vi "Generate Error.vi"(8 "Error In":errorcluster, 9 "Args":string[](array[string]), 10 "Nest Error":T1) -> (0 "Error Out":errorcluster)   [LabVIEW 2013, in "LVH-Nest.lvlib"]
uses:
  LVH-Nest.lvlib
  Type Defs/Nest Error.ctl
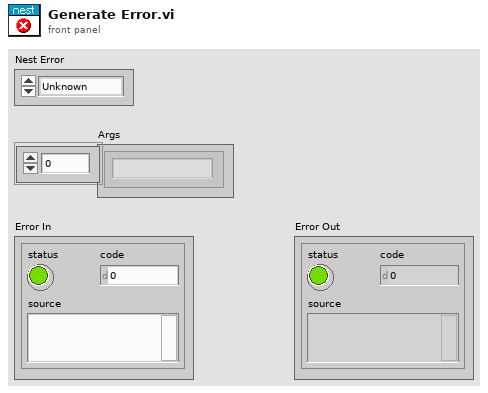
[diagram p1: front panel]
types:
  T1 = typedef "LVH-Nest.lvlib/Nest Error.ctl" = enum16{"Unknown", "Auth", "Read", "Invalid Structure Name", "Invalid Device Name", "Set Temp"}
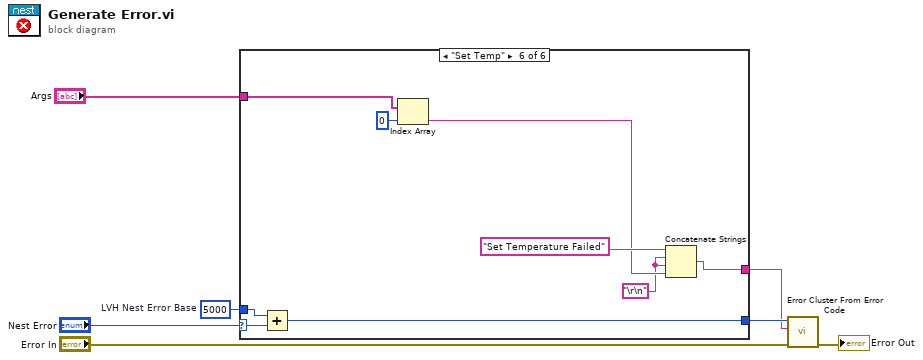
[diagram p0: block diagram]
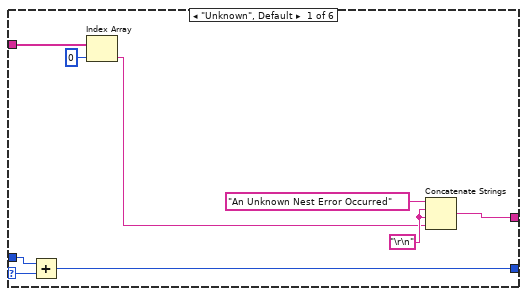
[diagram p2: hidden frame]
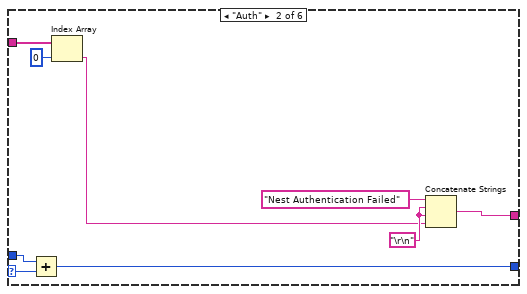
[diagram p3: hidden frame]
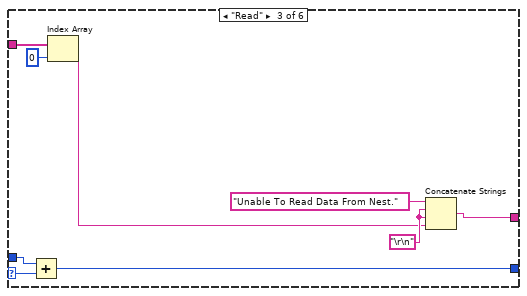
[diagram p4: hidden frame]
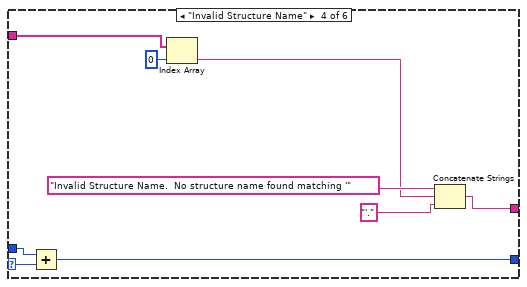
[diagram p5: hidden frame]
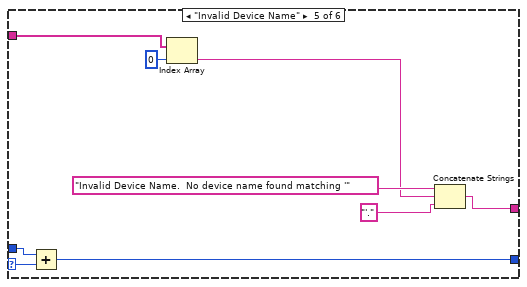
[diagram p6: hidden frame]
diagram:
  w5 = 5000  # LVH Nest Error Base
  n1 = case shown="\"Set Temp\"" "Nest Error" {
    selector: "Nest Error" -> [w16 w25 w34 w43 w52 w61]
    tunnel: [w15 w24 w33 w42 w51 w60] -> w7
    tunnel: [w14 w23 w32 w35 w44 w55] -> w6
    tunnel: w5 -> [w13 w22 w31 w41 w50 w59]
    tunnel: "Args" -> [w9 w18 w27 w39 w48 w57]
    frame "Unknown", Default {
      w11 = "\r\n"
      n2 = Add(x=w13, y=w16) -> (x+y=w15:i32)
      n3 = Index Array(array=w9, index=0) -> (element=w8:string)
      n4 = Concatenate Strings("An Unknown Nest Error Occurred" ("search string/char (-)"), w11, w11, w8) -> (w14:string)
    }
    frame "Auth" {
      w21 = "\r\n"
      n5 = Add(x=w22, y=w25) -> (x+y=w24:i32)
      n6 = Index Array(array=w18, index=0) -> (element=w17:string)
      n7 = Concatenate Strings("Nest Authentication Failed" ("search string/char (-)"), w21, w21, w17) -> (w23:string)
    }
    frame "Read" {
      w30 = "\r\n"
      n8 = Add(x=w31, y=w34) -> (x+y=w33:i32)
      n9 = Index Array(array=w27, index=0) -> (element=w26:string)
      n10 = Concatenate Strings("Unable To Read Data From Nest." ("search string/char (-)"), w30, w30, w26) -> (w32:string)
    }
    frame "Invalid Structure Name" {
      n11 = Add(x=w41, y=w43) -> (x+y=w42:i32)
      n12 = Index Array(array=w39, index=0) -> (element=w37:string)
      n13 = Concatenate Strings("Invalid Structure Name.  No structure name found matching '" ("search string/char (-)"), w37, "'." ("string")) -> (w35:string)
    }
    frame "Invalid Device Name" {
      n14 = Add(x=w50, y=w52) -> (x+y=w51:i32)
      n15 = Index Array(array=w48, index=0) -> (element=w46:string)
      n16 = Concatenate Strings("Invalid Device Name.  No device name found matching '" ("search string/char (-)"), w46, "'." ("string")) -> (w44:string)
    }
    frame "Set Temp" {
      w53 = "\r\n"
      n17 = Add(x=w59, y=w61) -> (x+y=w60:i32)
      n18 = Index Array(array=w57, index=0) -> (element=w54:string)
      n19 = Concatenate Strings("Set Temperature Failed" ("search string/char (-)"), w53, w53, w54) -> (w55:string)
    }
  }
  n20 = call <vilib>:"Error Cluster From Error Code.vi"("error in (no error)"="Error In", "error message (\"\")"=w6, "error code (0)"=w7) -> ("error out"=→"Error Out":errorcluster)  [unwired: 6 in]
